vi "AIT 664 Hardware Out Loop.vi"(0 "RT Data":T1 {"End System Handle" format="%x"; "Label Transfer Config"."Block Data Refs"."Data Reference" format="%.0x"; "Status Config"."Hardware Out Dur Reference" format="%.0x"; "Status Config"."Hardware In Dur Reference" format="%.0x"; "Status Config"."Hardware Out Count Reference" format="%.0x"; "Status Config"."Hardware In Count Reference" format="%.0x"; "Status Config"."Error Data Reference" format="%.0x"; "Hardware Output Tx Channels"."Message Settings"."Transmit Channel Data Reference" format="%.0x"; "Hardware Output Tx Channels"."Message Settings"."Queue Transmit Channel" format="%.0x"; "Hardware Output Tx Channels"."Message Settings"."Driver Data"."Num Bits" min=1 max=32; "Hardware Output Tx Channels"."Message Settings"."Block Data Refs"."Data Reference" format="%.0x"; "Hardware Output Tx Channels"."Rx Com Udp Port"."Handle" format="%08x"; "Hardware Output Tx Channels"."Tx Com Udp Port"."Handle" format="%08x"; "Hardware Input Rx Channels"."Message Settings"."Transmit Channel Data Reference" format="%.0x"; "Hardware Input Rx Channels"."Message Settings"."Queue Transmit Channel" format="%.0x"; "Hardware Input Rx Channels"."Message Settings"."Driver Data"."Num Bits" min=1 max=32; "Hardware Input Rx Channels"."Message Settings"."Block Data Refs"."Data Reference" format="%.0x"; "Hardware Input Rx Channels"."Rx Com Udp Port"."Handle" format="%08x"; "Hardware Input Rx Channels"."Tx Com Udp Port"."Handle" format="%08x"}, 5 "Channel Index":i32, 9 "Error Index":i32) -> ()   [LabVIEW 2013, in "AIT 664 Custom Device.lvlib"]
doc: "Given the loop rate by the user send data to the AIT 664 hardware.\n\nChannel Index - location in the hardware output tx channels array for this particular channel\nError Index - error fifo index"
uses:
  AIT 664 Custom Device.lvlib
  RT Controls/AIT 664  - RT Data.ctl
  RT Controls/AIT 664 - RT Hardware Channel.ctl
  RT Controls/AIT 664 - RT Message Settings.ctl
  <vilib>/NI Veristand/Custom Device API/Block Data Reference.ctl
  <vilib>/NI Veristand/Custom Device API/Data Reference.ctl
  RT Controls/AIT 664 - Driver Data.ctl
  Controls and Global/Start Bit.ctl
  Controls and Global/Number of Bits.ctl
  <vilib>/NI Veristand/Custom Device API/Custom Device Item Ref.ctl
  <userlib>/ARINC 664/AIT 664 Controls/General/Message Port.ctl
  <userlib>/ARINC 664/AIT 664 Controls/General/Direction.ctl
  <userlib>/ARINC 664/AIT 664 Controls/General/Message Port Type.ctl
  System Explorer/Controls/664 - Sampling Type.ctl
  RT Controls/Status Channels Config.ctl
  RT Controls/FIFO.ctl
  RT Controls/Label Transfer Config.ctl
  <vilib>/Platform/TimedLoop/XDataNode/timing_clust.ctl
  <vilib>/Platform/TimedLoop/XDataNode/nitl_modes.ctl
  <vilib>/Platform/TimedLoop/XDataNode/wakeup.ctl
  RT Controls/ReadWrite Selector.ctl
  <vilib>/Platform/TimedLoop/XDataNode/XDataNode.xnode
  <vilib>/Platform/TimedLoop/XDataNode/XDNodeRunTimeDep.lvlib
  <vilib>/NI Veristand/Custom Device Tools/Custom Device Utility Library/Custom Device Utility Library.lvlib
  <vilib>/NI Veristand/Custom Device API/Custom Device API.lvlib
  <userlib>/ARINC 664/AIT 664 API.lvlib
panel:
  in  "stop":bool
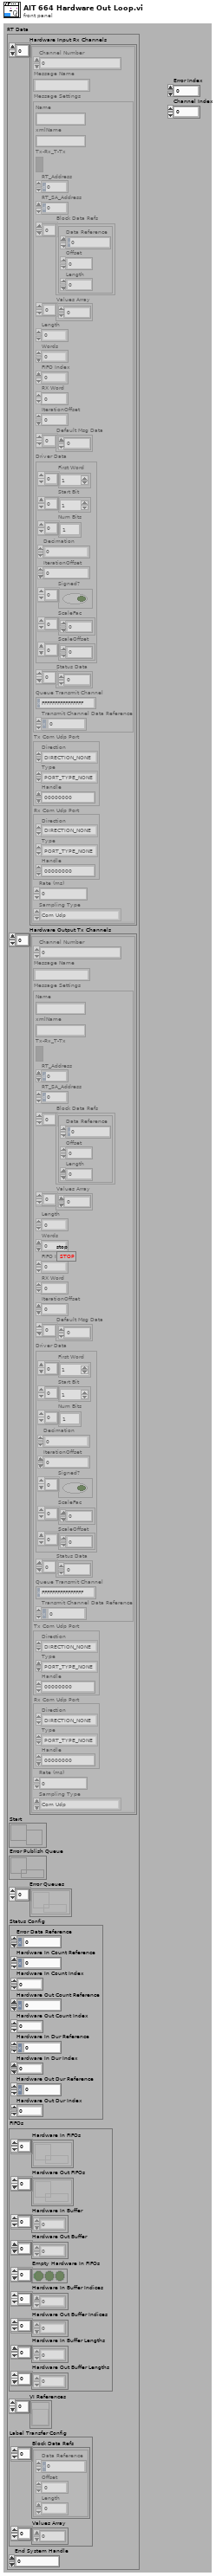
[diagram p1: front panel]
types:
  T1 = typedef "AIT 664 Custom Device.lvlib/AIT 664  - RT Data.ctl" = cluster{"Hardware Input Rx Channels":T2[], "Hardware Output Tx Channels":T2[], "Start":refnum<notifier>, "Error Publish Queue":refnum<queue>, "Error Queues":refnum<queue>[], "Status Config":T14, "FIFOs":T15, "VI References":refnum<vi>[], "Label Transfer Config":T16, "End System Handle ":u64}
  T2 = typedef "AIT 664 Custom Device.lvlib/AIT 664 - RT Hardware Channel.ctl" = cluster{"Channel Number":u16, "Message Name":string, "Message Settings":T3, "Tx Com Udp Port":T10, "Rx Com Udp Port":T10, "Rate (ms)":u32, "Sampling Type":T13}
  T3 = typedef "AIT 664 Custom Device.lvlib/AIT 664 - RT Message Settings.ctl" = cluster{"Name":string, "xmlName":string, "Tx-Rx_T-Tx":bool, "RT_Address":u8, "RT_SA_Address":u8, "Block Data Refs":T4[], "Values Array":dbl[], "Length":i32, "Words":i32, "FIFO Index":i32, "RX Word":u32, "IterationOffset":i32, "Default Msg Data":u8[], "Driver Data":T6, "Status Data":u32[], "Queue Transmit Channel":T9, "Transmit Channel Data Reference":T5}
  T4 = typedef "Custom Device API.lvlib/Block Data Reference.ctl" = cluster{"Data Reference":T5, "Offset":i32, "Length":i32}
  T5 = typedef "Custom Device API.lvlib/Data Reference.ctl" = i32
  T6 = typedef "AIT 664 Custom Device.lvlib/AIT 664 - Driver Data.ctl" = cluster{"First Word":T7[], "Start Bit":T7[], "Num Bits":T8[], "Decimation":i32, "IterationOffset":i32, "Signed?":bool[], "ScaleFac":dbl[], "ScaleOffset":dbl[]}
  T7 = typedef "AIT 664 Custom Device.lvlib/Start Bit.ctl" = i32
  T8 = typedef "AIT 664 Custom Device.lvlib/Number of Bits.ctl" = i32
  T9 = typedef "Custom Device API.lvlib/Custom Device Item Ref.ctl" = u64
  T10 = typedef "AIT 664 API.lvlib/Message Port.ctl" = cluster{"Direction":T11, "Type":T12, "Handle":u64}
  T11 = typedef "AIT 664 API.lvlib/Direction.ctl" = enum16{"DIRECTION_NONE", "DIRECTION_TX", "DIRECTION_RX"}
  T12 = typedef "AIT 664 API.lvlib/Message Port Type.ctl" = enum16{"PORT_TYPE_NONE", "COM_UDP", "SAP_UDP", "SAP_IP", "SAP_MAC", "COTS_MAC", "COTS_MAC_RAW"}
  T13 = typedef "AIT 664 Custom Device.lvlib/664 - Sampling Type.ctl" = enum16{"Com Udp", "Com Udp Queuing", "Sap Udp", "Sap Ip", "Sap Mac", "Unknown"}
  T14 = typedef "AIT 664 Custom Device.lvlib/Status Channels Config.ctl" = cluster{"Error Data Reference":T5, "Hardware In Count Reference":T5, "Hardware In Count Index":i32, "Hardware Out Count Reference":T5, "Hardware Out Count Index":i32, "Hardware In Dur Reference":T5, "Hardware In Dur Index":i32, "Hardware Out Dur Reference":T5, "Hardware Out Dur Index":i32}
  T15 = typedef "AIT 664 Custom Device.lvlib/FIFO.ctl" = cluster{"Hardware In FIFOs":refnum<k33>[], "Hardware Out FIFOs":refnum<k33>[], "Hardware In Buffer":dbl[], "Hardware Out Buffer":dbl[], "Empty Hardware In FIFOs":bool[], "Hardware In Buffer Indices":i32[], "Hardware Out Buffer Indices":i32[], "Hardware In Buffer Lengths":i32[], "Hardware Out Buffer Lengths":i32[]}
  T16 = typedef "AIT 664 Custom Device.lvlib/Label Transfer Config.ctl" = cluster{"Block Data Refs":T4[], "Values Array":dbl[]}
  T17 = typedef "AIT 664 Custom Device.lvlib/ReadWrite Selector.ctl" = enum16{"Inline Read", "Inline Write", "Async HWIn", "Async HWOut"}
  T18 = typedef "XDNodeRunTimeDep.lvlib/timing_clust.ctl" = cluster{"Expected End [f-1]":u64, "Actual End [f-1]":u64, "Finished Late? [f-1]":bool, "Expected End [i-1]":u64, "Actual End [i-1]":u64, "Finished Late? [i-1]":bool, "Expected Start [i]":u64, "Actual Start [i]":u64, "Expected Start [f]":u64, "Actual Start [f]":u64, "Source Name":string, "Structure Name":string, "Period":i64, "Deadline":i64, "Offset":i64, "Start":i64, "Priority":i32, "Timeout":i32, "Mode":T19, "Wakeup Reason":T20, "Error":errorcluster, "Source Type":string, "Secondary Source Type":string, "Global End Time":u64, "Global Start Time":u64, "Frame Duration":u64, "Iteration Duration":u64, "Assigned CPU":i32, "I/O Scan Engine Mode":u32}
  T19 = typedef "XDNodeRunTimeDep.lvlib/nitl_modes.ctl" = enum32{"No Change", "Process missed periods, maintain original phase", "Discard missed periods, maintain original phase", "Process missed periods, ignore original phase", "Discard missed periods, ignore original phase"}
  T20 = typedef "XDNodeRunTimeDep.lvlib/wakeup.ctl" = enum32{"Normal", "Aborted", "Asynchronous wakeup", "Timing source error", "Timed loop error", "Timeout"}
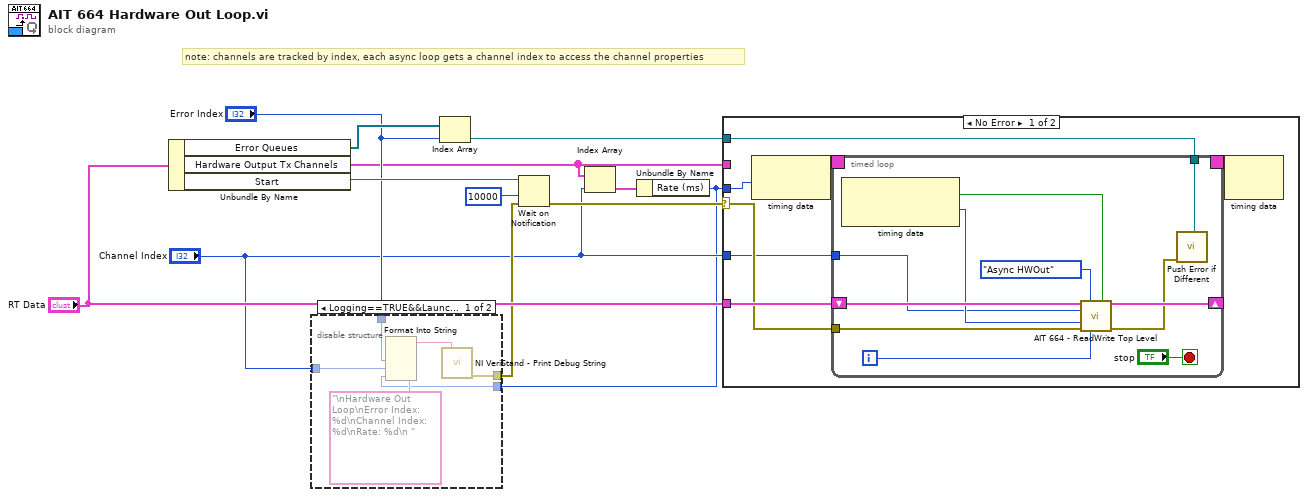
[diagram p0: block diagram]
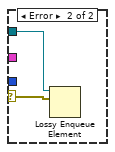
[diagram p2: hidden frame]
diagram:
  # "note: channels are tracked by index, each async loop gets a channel index to access the channel properties"
  n1 = Unbundle By Name("RT Data") -> ("Error Queues"=w9:refnum<queue>[], "Hardware Output Tx Channels"=w4:T2[], "Start"=w12:refnum<notifier>)
  n2 = Index Array(array=w9, index="Error Index") -> (element=w8:refnum<queue>)
  n3 = Index Array(array=w4, index="Channel Index") -> (element=w3:T2)
  n4 = Unbundle By Name(w3) -> ("Rate (ms)"=w1:u32)
  n5 = disable-structure shown="Logging==TRUE&&LaunchLoopLogging==TRUE" {
    disable-tunnel: "Error Index" -> [w17 _]
    disable-tunnel: [w15 _] -> w6
    disable-tunnel: "Channel Index" -> [w14 _]
    disable-tunnel: w1 -> [w13 _]
    frame condition #0 {
      n6 = Format Into String(format string="\nHardware Out Loop\nError Index: %d\nChannel Index: %d\nRate: %d\n ", w17, w14, w13) -> (resulting string=w16:string)  [unwired: 2 in, 1 out]
      n7 = call <vilib>:"NI VeriStand - Print Debug String.vi"("Message"=w16) -> ("error out"=w15:errorcluster)  [unwired: 10 in]
    }
    frame condition #1 (active) {
    }
  }
  n8 = Wait on Notification(notifier=w12, timeout in ms (-1)=10000, error in (no error)=w6) -> (error out=w11:errorcluster)  [unwired: 1 in, 3 out]
  n9 = case shown="No Error" w11 {
    selector: w11 -> [w21 w46]
    tunnel: w4 -> [_ _]
    tunnel: "RT Data" -> [w23 _]
    tunnel: w8 -> [w22 w45]
    tunnel: w1 -> [w20 _]
    tunnel: "Channel Index" -> [w19 _]
    frame No Error {
      n10 = node-c288(w20) -> (w25:T18)
      n11 = timed-loop {
        timing: w25 -> [_]
        timing-out: [_] -> w24
        shift-right: [w34] -> _
        shift-left: w23 -> [w35]
        tunnel: w22 -> [w32]
        tunnel: w21 -> [w31]
        tunnel: w19 -> [w27]
        i -> [w28]
        stop <- "stop" stop-if-true
        n12 = node-c288() -> (w30:bool, w29:i64)  [unwired: 1 in]
        n13 = call "AIT 664 - ReadWrite Top Level.vi"("RT Data in"=w35, "Mode"=ReadWrite_Selector."Async HWOut", "Late?"=w30, "Channel Index"=w27, "Iteration Duration"=w29, "error in (no error)"=w31, "Iteration"=w28) -> ("RT Data out"=w34:T1, "error out"=w33:errorcluster)  [unwired: 7 in]
        n14 = call "Push Error if Different.vi"("Error Queue"=w32, "error in"=w33) -> ()  [unwired: 14 in]
      }
      n15 = node-c288(w24) -> ()  [unwired: 1 out]
    }
    frame Error {
      n16 = Lossy Enqueue Element(queue=w45, element=w46) -> ()  [unwired: 1 in, 4 out]
    }
  }
